vi "AIResolution.vi"(9 "Polarity":enum16{"Unipolar", "Bipolar"}(ring)=enum."Bipolar", 10 "ADC Resolution":u32=12, 11 "Voltage Range":dbl=5.0) -> (3 "Voltage Resolution":dbl format="%#_6p")   [LabVIEW 2014]
doc: "Calculate the bin size, aka voltage resolution, given the working range, ADC resolution in bits, and polarity"
panel:
  # "Calculate the bin size, aka voltage resolution, given the working range, ADC resolution in bits, and polarity."
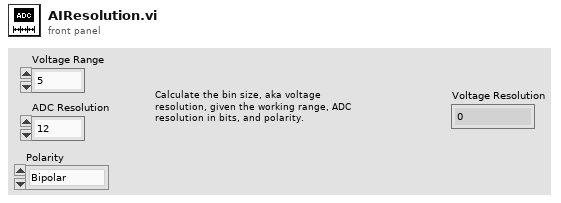
[diagram p1: front panel]
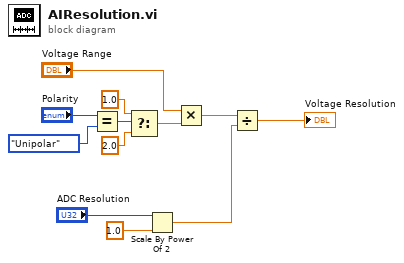
[diagram p0: block diagram]
diagram:
  n1 = Equal?(x="Polarity", y=enum16{"Unipolar", "Bipolar"}."Unipolar") -> (x = y?=w10:bool)
  n2 = Select(t=1.0, s=w10, f=2.0) -> (s? t:f=w7:dbl)
  n3 = Scale By Power Of 2(n="ADC Resolution", x=1.0) -> (x*2^n=w3:dbl)
  n4 = Multiply(x="Voltage Range", y=w7) -> (x*y=w2:dbl)
  n5 = Divide(x=w2, y=w3) -> (x/y=→"Voltage Resolution":dbl)
